vi "DataWrapper.vi"(0 "Device in":refnum<class "Device.lvclass">, 1 "Source":string, 2 "Description":string, 3 "Destination":string, 4 "value":variant, 5 "error in (no error)":errorcluster) -> (14 "Device out":refnum<class "Device.lvclass">, 15 "DataExchange":T1, 19 "error out":errorcluster)   [LabVIEW 2020, in "Device.lvlib" / "Device.lvclass"]
uses:
  Device.lvclass
  DataExchange.ctl
  Interface/DataListener/DataListener.lvclass
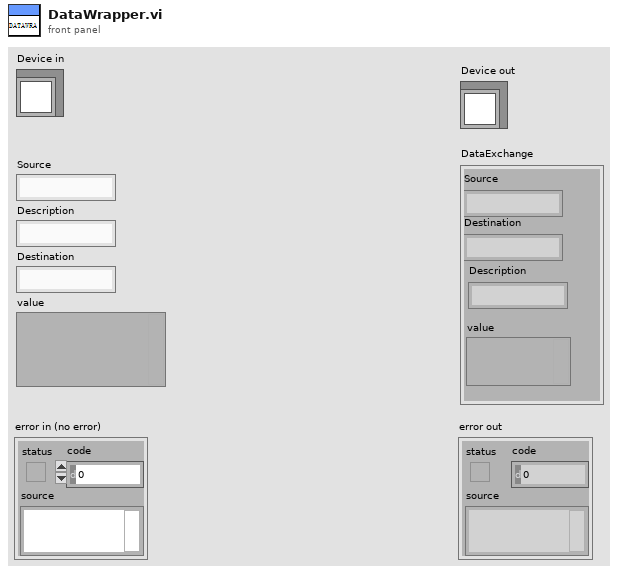
[diagram p1: front panel]
types:
  T1 = typedef "DataListener.lvclass/DataExchange.ctl" = cluster{"Source":string, "Destination":string, "Description":string, "value":variant}
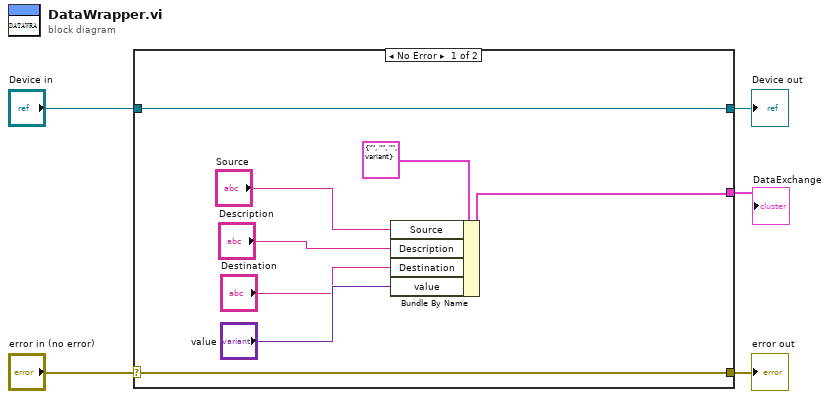
[diagram p0: block diagram]
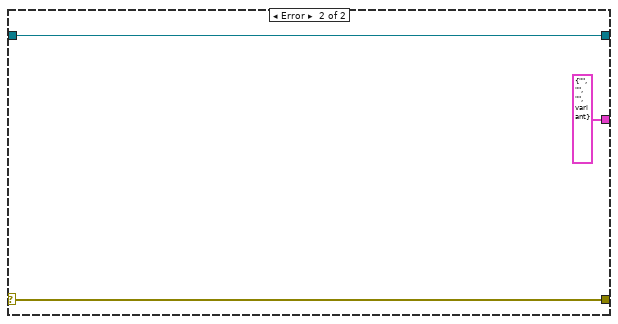
[diagram p2: hidden frame]
diagram:
  n1 = case shown="No Error" "error in (no error)" {
    selector: "error in (no error)" -> [w12 w16]
    tunnel: [w12 w16] -> w4
    tunnel: [w13 w15] -> w2
    tunnel: "Device in" -> [w13 w15]
    tunnel: [w11 T1 {"Source"="", "Destination"="", "Description"="", "value"=variant} ("DataExchange")] -> w1
    frame No Error {
      n2 = Bundle By Name(cluster=T1 {"Source"="", "Destination"="", "Description"="", "value"=variant} ("DataExchange"), "Source"="Source", "Description"="Description", "Destination"="Destination", "value"="value") -> (w11:T1)
    }
    frame Error {
    }
  }
  "error out" <- w4
  "Device out" <- w2
  "DataExchange" <- w1
